vi "subFormSourcePaths.vi"(0 "Repo Top-level":path, 11 "error in (no error)":errorcluster) -> (3 "Documentation Source Path":path, 4 "GACUtilityPaths":path[](array[path])=[path "C:/Users/admin/Documents/github/NIVeristandAdd-ons/VeriStand-steps-for-TestStand/Source/Source/CSharp/AddRemoveGACUtils/RemoveFromGAC.exe", path "C:/Users/admin/Documents/github/NIVeristandAdd-ons/VeriStand-steps-for-TestStand/Source/Source/CSharp/AddRemoveGACUtils/InstallToGAC.exe"], 6 "CSharp Assembly Project Path":path=path "C:/Users/admin/Documents/github/NIVeristandAdd-ons/VeriStand-steps-for-TestStand/Source/Source/CSharp/VeristandStepsAssembly/OpenWorkspaceDialog/VeristandSteps.csproj", 8 "TypePalette File Path":path=path "C:/Users/admin/Documents/github/NIVeristandAdd-ons/VeriStand-steps-for-TestStand/Source/Source/CustomPaletteFile/NI_VeristandTypes.ini", 10 "Icon File Path":path=path "C:/Users/admin/Documents/github/NIVeristandAdd-ons/VeriStand-steps-for-TestStand/Source/Source/CustomPaletteFile/Veristand_icon_vista.ico", 15 "error out":errorcluster)   [LabVIEW 2015, in "veristand-steps-build-tools.lvlib"]
uses:
  veristand-steps-build-tools.lvlib
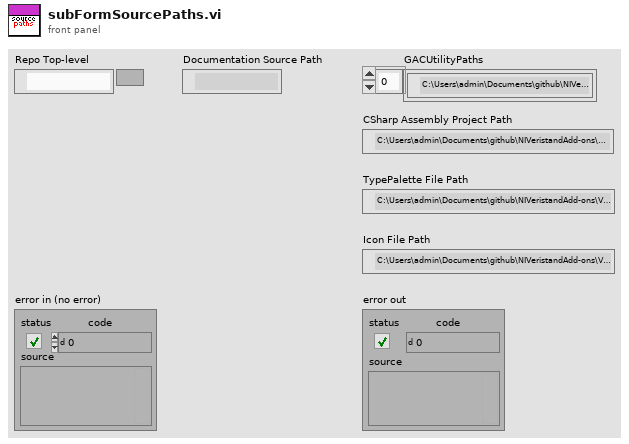
[diagram p1: front panel]
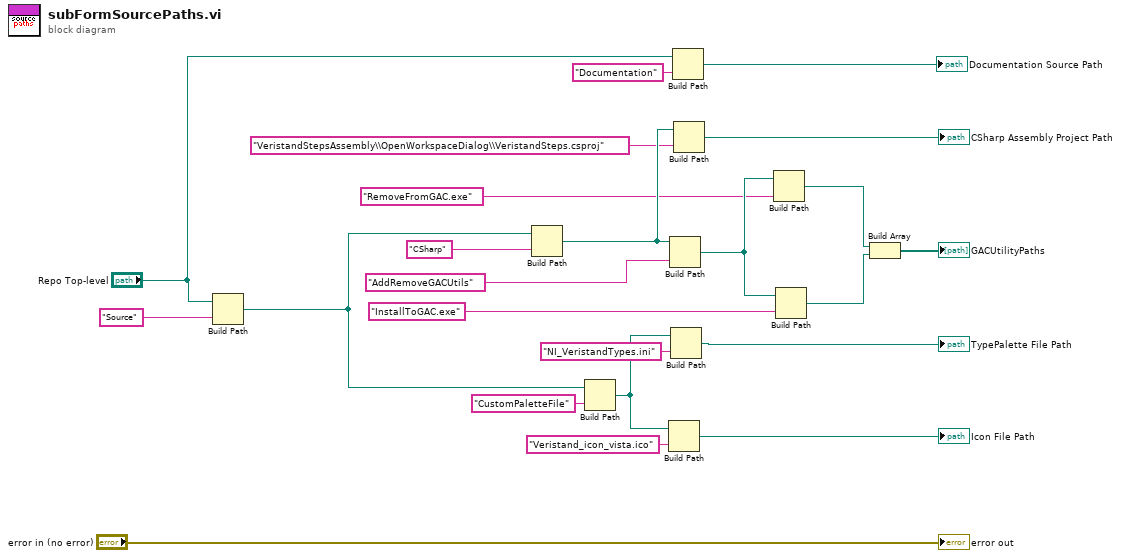
[diagram p0: block diagram]
diagram:
  n1 = Build Path(base path="Repo Top-level", name or relative path="Source") -> (appended path=w9:path)
  n2 = Build Path(base path=w9, name or relative path="CSharp") -> (appended path=w19:path)
  n3 = Build Path(base path=w9, name or relative path="CustomPaletteFile") -> (appended path=w21:path)
  n4 = Build Path(base path=w21, name or relative path="Veristand_icon_vista.ico") -> (appended path=→"Icon File Path":path)
  n5 = Build Path(base path=w19, name or relative path="AddRemoveGACUtils") -> (appended path=w16:path)
  n6 = Build Path(base path=w21, name or relative path="NI_VeristandTypes.ini") -> (appended path=→"TypePalette File Path":path)
  n7 = Build Path(base path="Repo Top-level", name or relative path="Documentation") -> (appended path=→"Documentation Source Path":path)
  n8 = Build Path(base path=w19, name or relative path="VeristandStepsAssembly\\OpenWorkspaceDialog\\VeristandSteps.csproj") -> (appended path=→"CSharp Assembly Project Path":path)
  n9 = Build Path(base path=w16, name or relative path="RemoveFromGAC.exe") -> (appended path=w13:path)
  n10 = Build Path(base path=w16, name or relative path="InstallToGAC.exe") -> (appended path=w12:path)
  n11 = Build Array(w13, w12) -> (→"GACUtilityPaths":path[])
  "error out" <- "error in (no error)"
